vi "Read Slew rate.vi"(0 "Source Mode":T1 items=["DC Voltage", "DC Current"], 11 "error in (no error)":errorcluster) -> (4 "Min Change":dbl, 15 "error out":errorcluster)   [LabVIEW 2024, in "devicePowerSequencerCoreLogic.lvlib"]
uses:
  devicePowerSequencerCoreLogic.lvlib
  controls/Source Mode.ctl
  Device Power Sequencer.lvlib
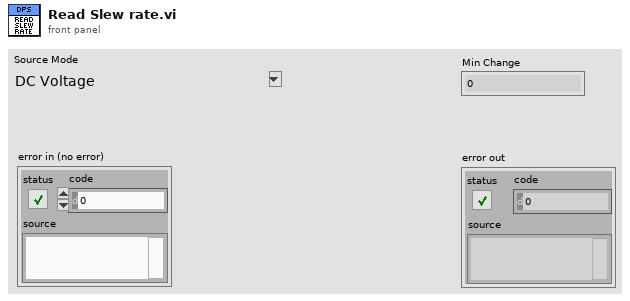
[diagram p1: front panel]
types:
  T1 = typedef "Device Power Sequencer.lvlib/Source Mode.ctl" = i32
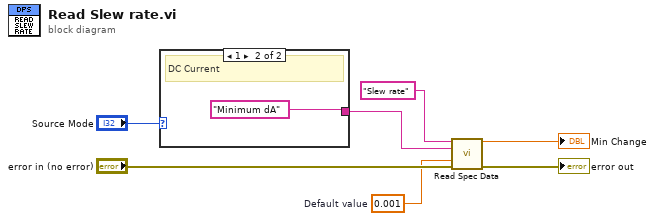
[diagram p0: block diagram]
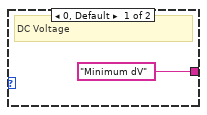
[diagram p2: hidden frame]
diagram:
  w1 = 0.001  # Default value
  n1 = case shown="1" "Source Mode" {
    tunnel: ["Minimum dV" ("section") "Minimum dA" ("section")] -> w3
    frame 0, Default {
      # "DC Voltage"
    }
    frame 1 {
      # "DC Current"
    }
  }
  n2 = call "Read Spec Data.vi"("section"="Slew rate", "key"=w3, "default value"=w1, "error in (no error)"="error in (no error)") -> ("value"=→"Min Change":dbl, "error out"=→"error out":errorcluster)  [unwired: 10 in]
